vi "Test Using data Generated in Setup.vi"(8 "error in (no error)":errorcluster, 11 "Dummy In":refnum<class "Example Test Case.lvclass">) -> (0 "error out":errorcluster, 3 "Dummy Out":refnum<class "Example Test Case.lvclass">)   [LabVIEW 2020, in "Example Test Case.lvclass"]
doc: "Test case demonstrating how to use data passed from setup method."
uses:
  Example Test Case.lvclass
  C:/git/astemes-lunit/source/API/LUnit Test Case/LUnit Test Case.lvclass
  Example Test Case.lvclass/Example Test Case.ctl
  Core/LUnit Test Case/LUnit Test Case.lvclass/LUnit Test Case.ctl
  b6345112-b2e7-4a25-94ce-86fe61bfcaf7.vi
  Core/LUnit Test Case/Private/Append Pass Result.vi
  Core/LUnit Test Case/Private/Append Fail Result.vi
  b6345112-b2e7-4a25-94ce-86fe61bfcaf7.vi/9c5d11cd-9439-4240-a1ee-d9baace9c924.vi
  Core/LUnit Test Case/Private/Run In UI.vi
  <vilib>/Utility/error.llb/Clear Errors.vi
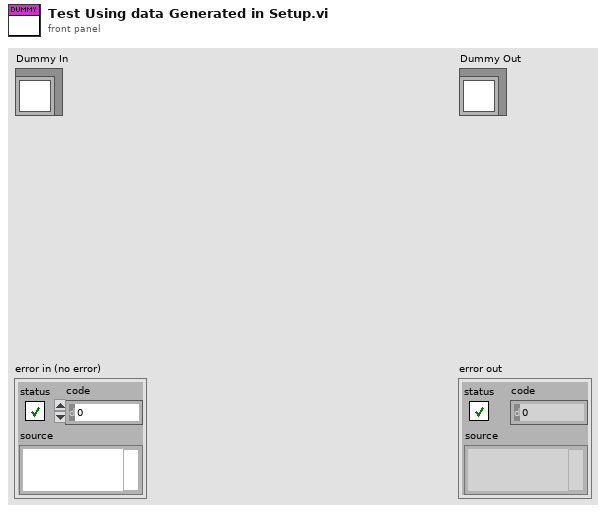
[diagram p1: front panel]
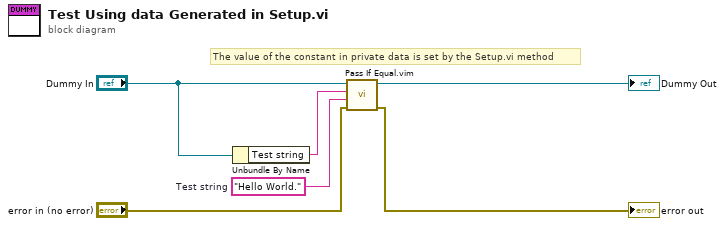
[diagram p0: block diagram]
diagram:
  w1 = "Hello World."  # Test string
  # "The value of the constant in private data is set by the Setup.vi method"
  n1 = Unbundle By Name("Dummy In") -> ("Test string"=w2:string)
  n2 = call "Pass If Equal.vim"("error in (no error)"="error in (no error)", "Actual"=w1, "Expected"=w2, "LUnit Test Case In"="Dummy In") -> ("error out"=→"error out":errorcluster, "LUnit Test Case Out"=→"Dummy Out":refnum<class "Example Test Case.lvclass">)  [unwired: 6 in]
